vi "OAT Orbit Plot Indicator.vi"() -> ()   [LabVIEW 2017]
doc: "Uses the Orbit Plot to display the the dynamic motion of the center of the shaft on a customized XY graph."
uses:
  <vilib>/addons/Sound and Vibration/Order Analysis/Backward Compatibility/SubVIs/oa_Orbit Plot Control.ctl
  <vilib>/addons/Sound and Vibration/Order Analysis/Backward Compatibility/OAT Orbit Plot (Unfiltered).vi
panel:
  out "orbit plot":T1
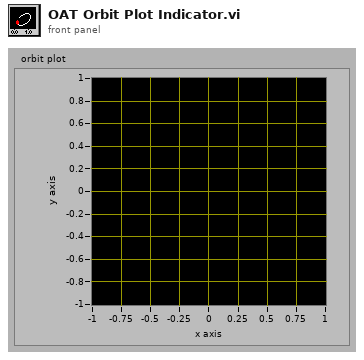
[diagram p1: front panel]
types:
  T1 = typedef "oa_Orbit Plot Control.ctl" = cluster{dbl[], dbl[]}[]
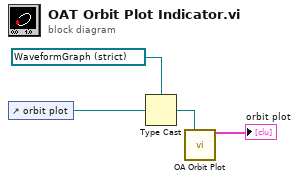
[diagram p0: block diagram]
diagram:
  n1 = control-ref of="orbit plot"() -> (w3:refnum<vi>)
  n2 = Type Cast(type=refnum<vi> refnum ("orbit plot ref"), x=w3) -> (*(type *) &x=w1:refnum<vi>)
  n3 = call-poly <vilib>:"OA Orbit Plot.vi"("orbit plot ref"=w1) -> ("orbit plot"=→"orbit plot":T1)  [unwired: 13 in, 1 out]
